vi "Cal IC (VIRef).vi"(8 "error in (no error)":errorcluster, 10 "IC in":variant, 11 "Domain_Evolut_2D_Rect in":refnum<class "NI_Domain_Evolut_2D_Rect.lvclass">) -> (0 "error out":errorcluster, 2 "IC out":variant, 3 "Domain_Evolut_2D_Rect out":refnum<class "NI_Domain_Evolut_2D_Rect.lvclass">)   [LabVIEW 2020, in "NI_PDE.lvlib" / "NI_Domain_Evolut_2D_Rect.lvclass"]
uses:
  <vilib>/gmath/pde.llb/DomainClass/Domain_Evolut_2D_Rect/NI_Domain_Evolut_2D_Rect.lvclass
  <vilib>/gmath/pde.llb/ICClass/IC_2D_VIRef/IC Data.ctl
  <vilib>/gmath/pde.llb/Common/PDE_IC Type.ctl
  <vilib>/gmath/pde.llb/ICClass/IC_2D_Numeric/IC Data.ctl
  <vilib>/gmath/pde.llb/DomainClass/Domain_Evolut_2D_Rect/NI_Domain_Evolut_2D_Rect.lvclass/NI_Domain_Evolut_2D_Rect.ctl
  <vilib>/Analysis/1siggen.llb/Ramp Pattern by Samples.vi
  <vilib>/gmath/NI_PDE.lvlib
  <vilib>/gmath/pde.llb/ICClass/IC_2D_Numeric/NI_IC_2D_Numeric.lvclass
  <vilib>/gmath/pde.llb/ICClass/IC_2D_VIRef/NI_IC_2D_VIRef.lvclass
  <vilib>/Analysis/NI_AALBase.lvlib
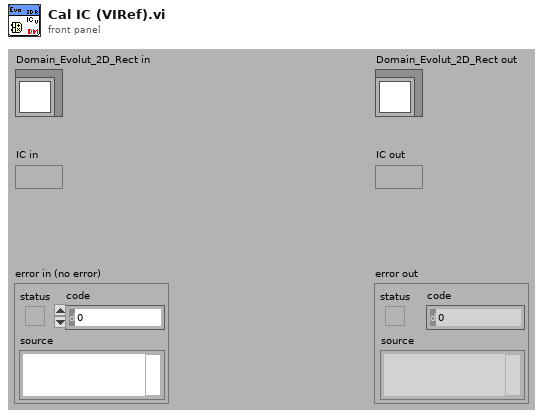
[diagram p1: front panel]
types:
  T1 = typedef "NI_PDE.lvlib/NI_IC_2D_Numeric.lvclass/IC Data.ctl" = cluster{"type":T2, "H":dbl[][]}
  T2 = typedef "NI_PDE.lvlib/PDE_IC Type.ctl" = i32
  T3 = typedef "NI_PDE.lvlib/NI_IC_2D_VIRef.lvclass/IC Data.ctl" = cluster{"type":T2, "H":refnum<vi>, "data":variant}
  T4 = cluster{"initial t":dbl, "final t":dbl, "# of t-points":i32}
  T5 = cluster{"start x":dbl, "end x":dbl, "# of x-points":i32}
  T6 = cluster{"start y":dbl, "end y":dbl, "# of y-points":i32}
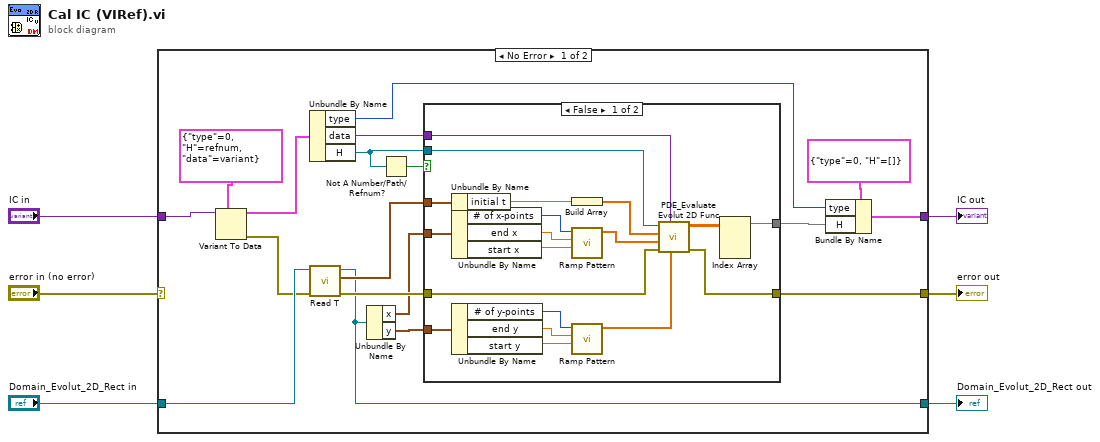
[diagram p0: block diagram]
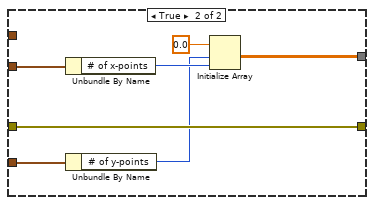
[diagram p2: hidden frame]
diagram:
  n1 = case shown="No Error" "error in (no error)" {
    selector: "error in (no error)" -> [_ w53]
    tunnel: "Domain_Evolut_2D_Rect in" -> [w13 w52]
    tunnel: [w9 w52] -> w6
    tunnel: [w14 w53] -> w5
    tunnel: [w22 w51] -> w2
    tunnel: "IC in" -> [w21 w51]
    frame No Error {
      n2 = Variant To Data(type=T3 {"type"=0, "H"=refnum, "data"=variant} ("IC data"), Variant=w21) -> (data=w17:T3, error out=w10:errorcluster)  [unwired: 1 in]
      n3 = Unbundle By Name(w17) -> ("type"=w16:T2, "data"=w20:variant, "H"=w19:refnum<vi>)
      n4 = call-dynamic "Read T.vi"("error in (no error)"=w10, "Domain_Evolut.lvclass in"=w13) -> ("error out"=w12:errorcluster, "t"=w11:T4, "Domain_Evolut.lvclass out"=w9:refnum<class "NI_Domain_Evolut_2D_Rect.lvclass">)  [unwired: 7 out]
      n5 = Unbundle By Name(w9) -> ("x"=w8:T5, "y"=w7:T6)
      n6 = Not A Number/Path/Refnum?(number/path/refnum=w19) -> (NaN/Path/Refnum?=w18:bool)
      n7 = case shown="False" w18 {
        tunnel: [w25 w50] -> w15
        tunnel: w11 -> [w43 _]
        tunnel: w12 -> [w39 w48]
        tunnel: [w42 w48] -> w14
        tunnel: w19 -> [w41 _]
        tunnel: w20 -> [w40 _]
        tunnel: w8 -> [w38 w47]
        tunnel: w7 -> [w30 w46]
        frame False {
          n8 = Unbundle By Name(w43) -> ("initial t"=w37:dbl)
          n9 = Unbundle By Name(w38) -> ("# of x-points"=w28:i32, "end x"=w35:dbl, "start x"=w34:dbl)
          n10 = Unbundle By Name(w30) -> ("# of y-points"=w27:i32, "end y"=w31:dbl, "start y"=w32:dbl)
          n11 = Build Array(w37) -> (w36:dbl[])
          n12 = call-poly <vilib>:"Ramp Pattern.vi"("start"=w34, "end"=w35, "samples"=w28) -> ("Ramp Pattern"=w33:dbl[])  [unwired: 7 in, 1 out]
          n13 = call-poly <vilib>:"Ramp Pattern.vi"("start"=w32, "end"=w31, "samples"=w27) -> ("Ramp Pattern"=w29:dbl[])  [unwired: 7 in, 1 out]
          n14 = call <vilib>:"PDE_Evaluate Evolut 2D Func.vi"("Y"=w29, "data"=w40, "error in (no error)"=w39, "X"=w33, "T"=w36, "VIRef"=w41) -> ("error out"=w42:errorcluster, "F(t, x, y)"=w26:dbl[][][])  [unwired: 4 out]
          n15 = Index Array(array=w26) -> (element=w25:dbl[][])  [unwired: 3 in]
        }
        frame True {
          n16 = Unbundle By Name(w47) -> ("# of x-points"=w45:i32)
          n17 = Unbundle By Name(w46) -> ("# of y-points"=w44:i32)
          n18 = Initialize Array(0.0 ("element"), w44, w45) -> (w50:dbl[][])
        }
      }
      n19 = Bundle By Name(cluster=T1 {"type"=0, "H"=[]} ("IC data"), "type"=w16, "H"=w15) -> (w22:T1)
    }
    frame Error {
    }
  }
  "Domain_Evolut_2D_Rect out" <- w6
  "error out" <- w5
  "IC out" <- w2
